vi "SIRWedge.vi"(8 "P":cluster{"x cm":dbl, "y cm":dbl, "z cm":dbl}={"x cm"=0.20000000000000018, "y cm"=-4.0, "z cm"=1.4} {"x cm" format="%.2f"; "z cm" format="%.2f"; "y cm" format="%.2f"}, 9 "Variables":T3={"sound spd (cm/s)"=150000, "time step (s)"=1e-08} {"time step (s)" format="%.2e"}, 11 "strip":T4={"Radius cm"=9.0, "h (cm)"=2.0, "a (cm)"=4.0} {"Radius cm" format="%.2f"; "a (cm)" format="%.2f"; "h (cm)" format="%.2f"}) -> (0 "r values (cm)":T1 {"r5" format="%.4f"; "r4" format="%.4f"; "r3" format="%.4f"; "r2" format="%.4f"; "r1" format="%.4f"; "r0" format="%.4f"}, 1 "h cap offset":dbl[](graph), 2 "h cap":dbl[](graph), 3 "h wedge":dbl[](graph), 4 "wedge delay":i32, 5 "Location Tests":T2, 6 "Case Number":i32, 7 "cap delay pts":i32)   [LabVIEW 2022 SP3]
uses:
  <vilib>/Utility/file.llb/Write To Spreadsheet File (DBL).vi
  <vilib>/Analysis/NI_AALBase.lvlib
panel:
  in  "Save":bool
  out "Waveform Graph":dbl[][](graph)
  in  "Norm hs":bool
  out "cap to wedge offset":i32
  in  "temp":bool
  # "in wedge"
  # "r5 good"
  # "in cap"
  # "r1 on wedge"
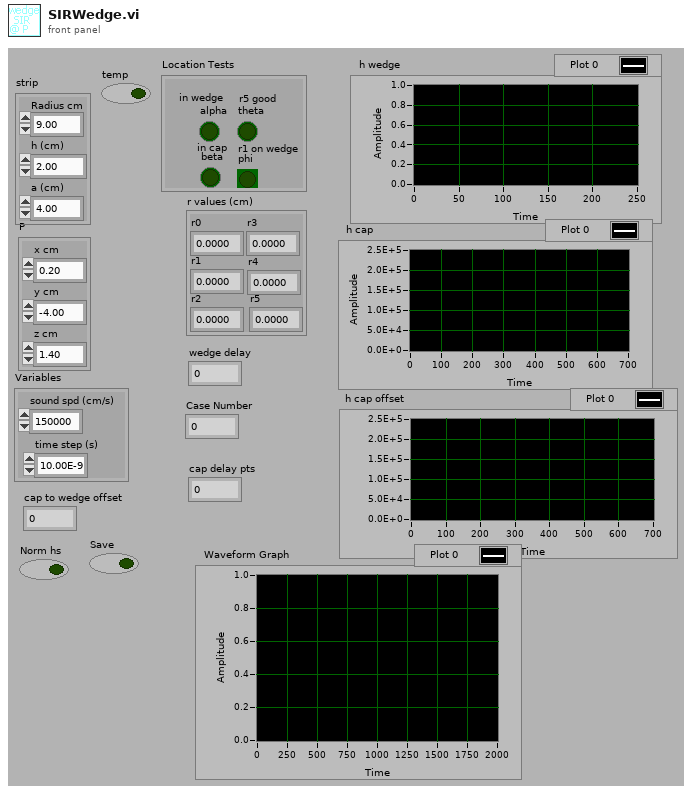
[diagram p1: front panel]
types:
  T1 = cluster{"r0":dbl, "r1":dbl, "r2":dbl, "r3":dbl, "r4":dbl, "r5":dbl}
  T2 = cluster{"alpha":bool, "beta":bool, "theta":bool, "phi":bool}
  T3 = cluster{"sound spd (cm/s)":i32, "time step (s)":sgl}
  T4 = cluster{"Radius cm":dbl, "h (cm)":dbl, "a (cm)":dbl}
  T5 = cluster{"r (cm)":dbl, "phih":dbl, "thetaw":dbl, "A":dbl, "B":dbl, "Dtemp":dbl}
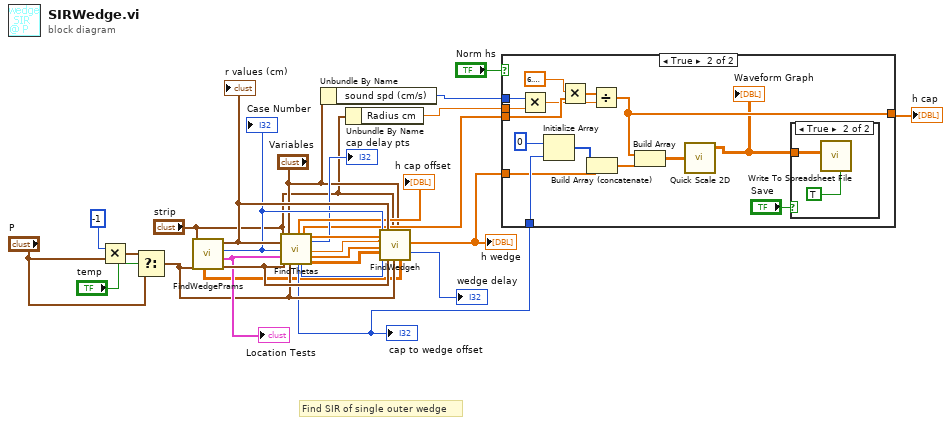
[diagram p0: block diagram]
diagram:
  # "Find SIR of single outer wedge"
  n1 = Multiply(x=-1, y="P") -> (x*y=w19:cluster{"x cm":dbl, "y cm":dbl, "z cm":dbl})
  n2 = Select(t=w19, s="temp", f="P") -> (s? t:f=w8:cluster{"x cm":dbl, "y cm":dbl, "z cm":dbl})
  n3 = call "FindWedgePrams.vi"("P"=w8, "strip"="strip") -> ("variables"=w25:T5, "Location Tests"=w21:T2, "Case Number"=w22:i32, "r values (cm)"=w26:T1, "Transform matrix"=w1:dbl[][])  [unwired: 2 out]
  "Case Number" <- w22
  "Location Tests" <- w21
  "r values (cm)" <- w26
  n4 = call "FindThetas.vi"("strip"="strip", "r values (cm)"=w26, "Case Number"=w22, "Location Tests"=w21, "P constants"=w25, "Variables"="Variables", "P (cm)"=w8) -> ("h(r,t) offset"=→"h cap offset":dbl[], "cap to wedge offset"=w4:i32, "h(r,t)"=w11:dbl[], "wedge delay pts"=w24:i32, "beta(t)/2"=w15:dbl[], "cap delay pts"=→"cap delay pts":i32, "rmin out"=w17:dbl, "sigma"=w27:dbl[], "slice coords"=w23:dbl[][])  [unwired: 4 out]
  "cap to wedge offset" <- w4
  n5 = Unbundle By Name("Variables") -> ("sound spd (cm/s)"=w9:i32)
  n6 = Unbundle By Name("strip") -> ("Radius cm"=w6:dbl)
  n7 = call "FindWedgeh.vi"("Case Number"=w22, "cap theta"=w15, "rmin out"=w17, "Sigma"=w27, "slice thetas"=w23, "slice delay points in"=w24, "r values"=w26, "P constants"=w25, "strip"="strip", "P"=w8, "Variables"="Variables", "Transform matrix"=w1) -> ("h wedge"=w3:dbl[], "slice delay out"=→"wedge delay":i32)  [unwired: 6 out]
  "h wedge" <- w3
  n8 = case shown="True" "Norm hs" {
    tunnel: w9 -> [_ w43]
    tunnel: w11 -> [w28 w40]
    tunnel: [w28 w34] -> w2
    tunnel: w6 -> [_ w42]
    tunnel: w4 -> [_ w36]
    tunnel: w3 -> [_ w33]
    frame False {
    }
    frame True {
      n9 = Multiply(x=w43, y=w42) -> (x*y=w38:dbl)
      n10 = Initialize Array(0, w36) -> (w32:i32[])
      n11 = Multiply(x=6.283185307179586, y=w40) -> (x*y=w39:dbl[])
      n12 = Build Array (concatenate)(w32, w33) -> (w35:dbl[])
      n13 = Divide(x=w39, y=w38) -> (x/y=w34:dbl[])
      n14 = Build Array(w34, w35) -> (w30:dbl[][])
      n15 = call <vilib>:"Quick Scale 2D.vi"("X"=w30) -> ("Yij=Xij/Max|X|"=w29:dbl[][])  [unwired: 2 out]
      "Waveform Graph" <- w29
      n16 = case shown="True" "Save" {
        tunnel: w29 -> [_ w44]
        frame False {
        }
        frame True {
          n17 = call-poly <vilib>:"Write To Spreadsheet File.vi"("transpose? (no:F)"=TRUE, "2D data"=w44) -> ()  [unwired: 4 in, 3 out]
        }
      }
    }
  }
  "h cap" <- w2
